vi "SVL RMS Level.vi"   [LabVIEW 2017, in "SoundVib_VibrationLevel.lvlib"]
doc: "Computes the root-mean-square (RMS) level of <B>scaled signal [EU]</B> or <B>even-angle signal [EU]</B>. <B>Scaled signal [EU]</B> should have a zero DC component. You can attenuate the DC component with hardware AC-coupling filters and with software high-pass filters. Wire data to the <B>scaled signal [EU]</B> input to determine the polymorphic instance to use or manually select the instance."
uses:
  <vilib>/addons/Sound and Vibration/svt_Level/SoundVib_VibrationLevel.lvlib
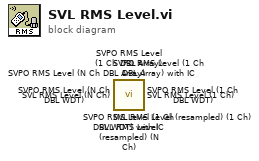
[diagram p0: block diagram]
diagram:
  n1 = call <vilib>:"SVPO RMS Level (1 Ch DBL WDT) with IC.vi"() -> ()  [unwired: 8 in, 4 out]
  n2 = call <vilib>:"SVPO RMS Level (1 Ch DBL Array) with IC.vi"() -> ()  [unwired: 9 in, 3 out]
  n3 = call <vilib>:"SVPO RMS Level (N Ch DBL WDT).vi"() -> ()  [unwired: 9 in, 3 out]
  n4 = call <vilib>:"SVPO RMS Level (1 Ch DBL WDT).vi"() -> ()  [unwired: 9 in, 3 out]
  n5 = call <vilib>:"SVPO RMS Level (N Ch DBL Array).vi"() -> ()  [unwired: 10 in, 2 out]
  n6 = call <vilib>:"SVPO RMS Level (1 Ch DBL Array).vi"() -> ()  [unwired: 10 in, 2 out]
  n7 = call <vilib>:"SVL RMS Level (resampled) (N Ch).vi"() -> ()  [unwired: 9 in, 3 out]
  n8 = call <vilib>:"SVL RMS Level (resampled) (1 Ch).vi"() -> ()  [unwired: 9 in, 3 out]
  n9 = call <vilib>:"SVL RMS Level (N Ch).vi"() -> ()  [unwired: 9 in, 3 out]
  n10 = call <vilib>:"SVL RMS Level (1 Ch).vi"() -> ()  [unwired: 9 in, 3 out]
